vi "1 bit transfert.vi"(1 "Min time SCL low (uSec)":u32, 2 "Min Time SCL high (uSec)":u32, 3 "Data bit":bool) -> ()   [LabVIEW 2013]
uses:
  <vilib>/rvi/eio/common/nirviEmuTemplateMethod_errors.vi
  <vilib>/eio/EIONode/EIONode.xnode
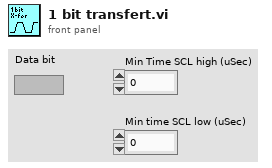
[diagram p1: front panel]
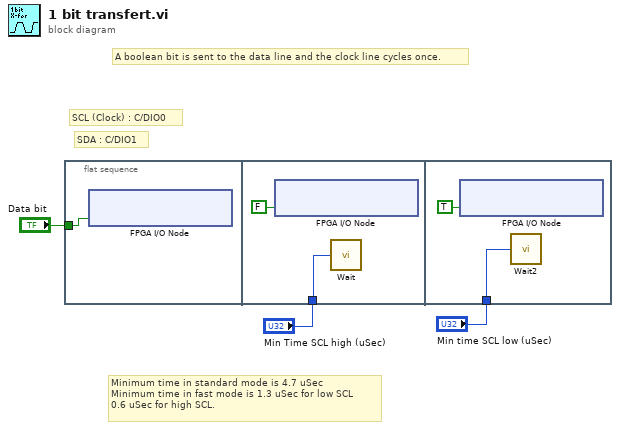
[diagram p0: block diagram]
diagram:
  # "A boolean bit is sent to the data line and the clock line cycles once."
  # "Minimum time in standard mode is 4.7 uSec\nMinimum time in fast mode is 1.3 uSec for low SCL\n0.6 uSec for high SCL."
  # "SDA : C/DIO1"
  # "SCL (Clock) : C/DIO0"
  n1 = flat-sequence {
    tunnel: "Data bit" -> [w4]
    tunnel: "Min Time SCL high (uSec)" -> [w6]
    tunnel: "Min time SCL low (uSec)" -> [w8]
    frame #0 {
      n2 = xnode "FPGA I/O Node"("ConnectorB/DIO13"=w4) -> ()  [unwired: 1 in, 1 out]
    }
    frame #1 {
      n3 = xnode "FPGA I/O Node"("ConnectorB/DIO12"=FALSE) -> ()  [unwired: 1 in, 1 out]
      n4 = call "Wait"("Count(uSec)"=w6) -> ()  [unwired: 1 out]
    }
    frame #2 {
      n5 = xnode "FPGA I/O Node"("ConnectorB/DIO12"=TRUE) -> ()  [unwired: 1 in, 1 out]
      n6 = call "Wait2"("Count(uSec)"=w8) -> ()  [unwired: 1 out]
    }
  }
